vi "RS NOR.vi"(1 "Reset":bool=TRUE, 2 "Set":bool=TRUE) -> (0 "Out":bool)   [LabVIEW 2016]
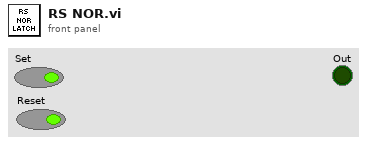
[diagram p1: front panel]
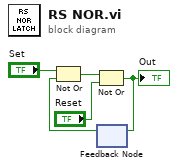
[diagram p0: block diagram]
diagram:
  n1 = feedback #1() -> (w1:bool)  [unwired: 1 in]
  n2 = Not Or(1:w1, 2:"Set") -> (0:w3:bool)
  n3 = Not Or(1:"Reset", 2:w3) -> (0:w2:bool)
  "Out" <- w2
  n4 = feedback-in #1(w2) -> ()
